vi "SetLocalSavingPath.vi"(8 "error in (no error)":errorcluster, 10 "Path in":path, 11 "Photometrics Cam v2 in":refnum<class "Photometrics_CH-250_Cam.lvclass">) -> (0 "error out":errorcluster, 2 "Path out":path, 3 "Photometrics Cam v2 out":refnum<class "Photometrics_CH-250_Cam.lvclass">)   [LabVIEW 2013, in "Photometrics_CH-250_Cam.lvclass"]
uses:
  Photometrics_CH-250_Cam.lvclass
  Photometrics_CH-250_Cam.lvclass/Photometrics_CH-250_Cam.ctl
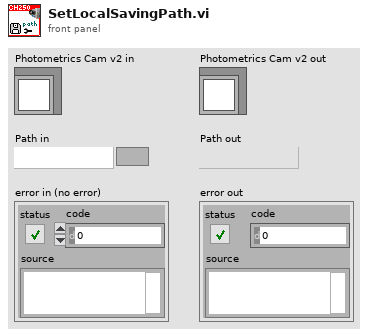
[diagram p1: front panel]
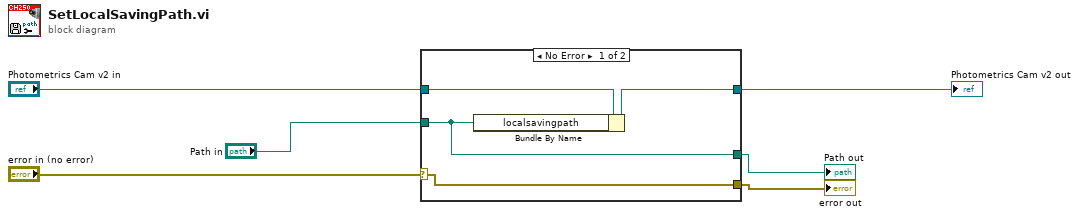
[diagram p0: block diagram]
diagram:
  n1 = case shown="No Error" "error in (no error)" {
    selector: "error in (no error)" -> [w8 w13]
    tunnel: [w10 w12] -> w1
    tunnel: "Photometrics Cam v2 in" -> [w9 w12]
    tunnel: "Path in" -> [w7 w11]
    tunnel: [w8 w13] -> w5
    tunnel: [w7 w11] -> w6
    frame No Error {
      n2 = Bundle By Name(cluster=w9, "localsavingpath"=w7) -> (w10:refnum<class "Photometrics_CH-250_Cam.lvclass">)
    }
    frame Error {
    }
  }
  "Path out" <- w6
  "error out" <- w5
  "Photometrics Cam v2 out" <- w1
